vi "DIV_ACELTRS..vi"(5 "LIMITE MIN 2":dbl, 6 "LIMITE MAX 2":dbl, 7 "all rows":dbl[][](array[numeric])) -> (0 "concatenated string":string, 1 "ACELEROMETROS OK":bool)   [LabVIEW 2015]
panel:
  out "spreadsheet string":string
  out "Array 6":string[](array[string])
  out "transposed array":string[][](array[string])
  out "Array 5":string[](array[string])
  out "Array 4":string[][](array[string])
  out "Array 3":string[][](array[string])
  out "deleted portion 4":i32
  out "Array 2":string[][](array[string])
  out "Array":string[](array[string])
  out "deleted portion 3":i32
  out "Array 8":string[][](array[string])
  out "repet":i32
  out "FALLO ACELEROMETROS":string[][](array[string])
  out "BAJA SEÑAL 2":bool
  out "ACEL.SATURADO 2":bool
  out "deleted portion 2":i32
  out "deleted portion":i32
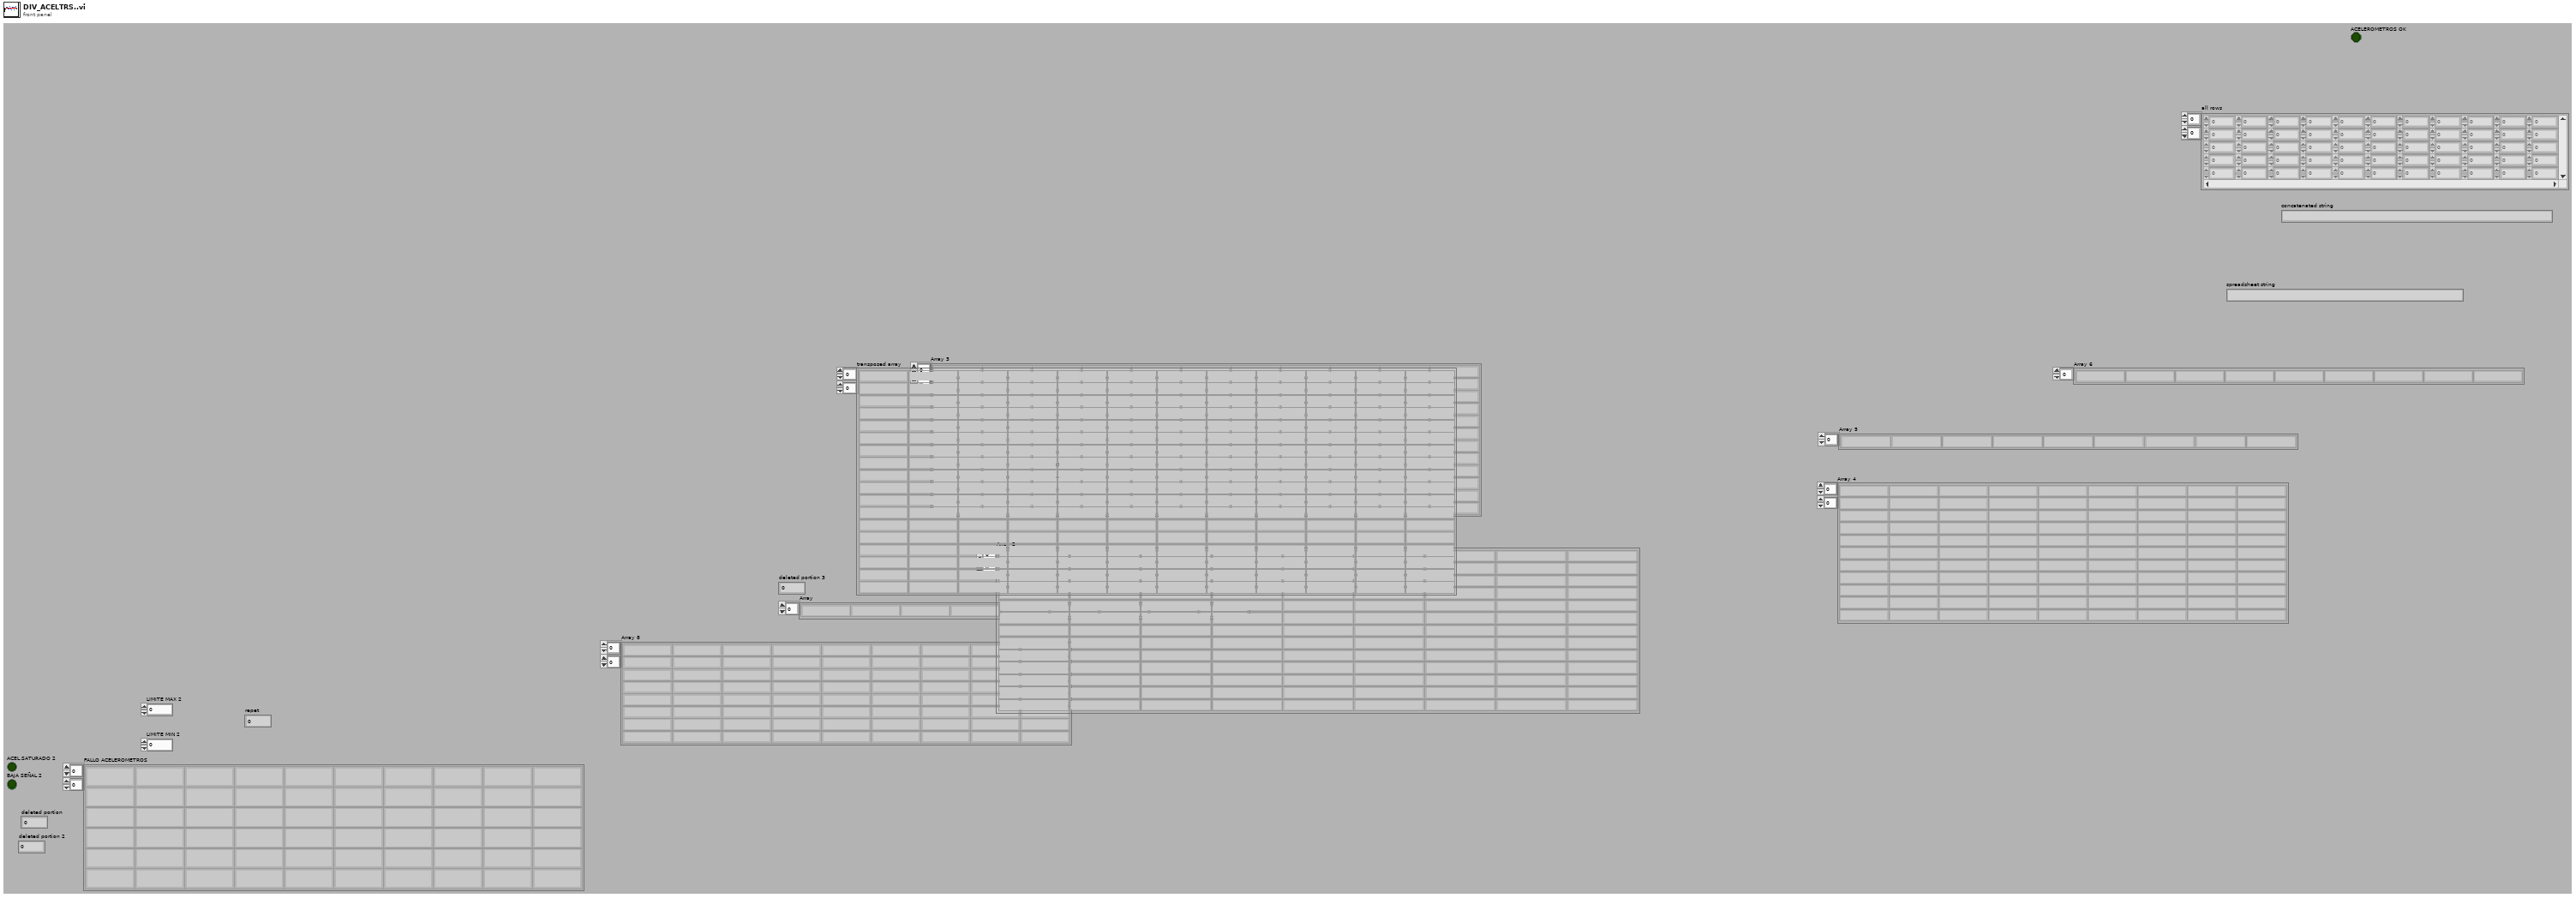
[diagram p1: front panel]
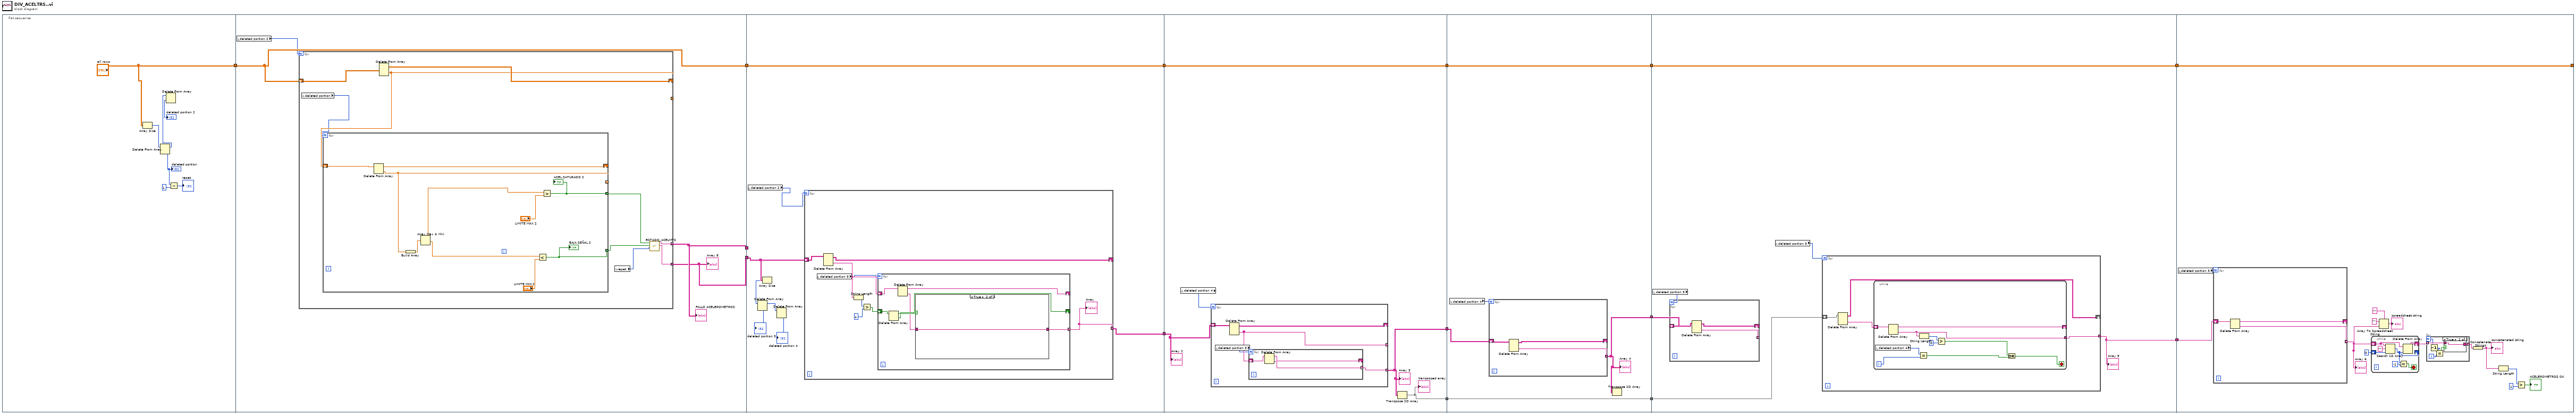
[diagram p0: block diagram]
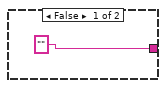
[diagram p2: hidden frame]
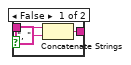
[diagram p3: hidden frame]
diagram:
  n1 = flat-sequence {
    tunnel: ["all rows"] -> w14
    tunnel: w14 -> [w25]
    tunnel: [w25] -> w13
    tunnel: [w23] -> w11
    tunnel: [w22] -> w10
    tunnel: w13 -> [w52]
    tunnel: [w52] -> w12
    tunnel: w11 -> [_]
    tunnel: w10 -> [w50]
    tunnel: [w47] -> w9
    tunnel: w12 -> [w74]
    tunnel: w9 -> [w73]
    tunnel: [w74] -> w8
    tunnel: [w71] -> w7
    tunnel: [w70] -> w3
    tunnel: w8 -> [w87]
    tunnel: w7 -> [w85]
    tunnel: [w87] -> w6
    tunnel: [w84] -> w5
    tunnel: [w83] -> w4
    tunnel: w3 -> [w83]
    tunnel: w6 -> [w96]
    tunnel: w5 -> [w94]
    tunnel: w4 -> [w92]
    tunnel: [w96] -> w2
    tunnel: [w91] -> w1
    tunnel: [w127] -> _
    tunnel: w2 -> [w127]
    tunnel: w1 -> [w125]
    frame #0 {
      n2 = Array Size(array="all rows") -> (size(s)=w21:i32[])
      n3 = Delete From Array(array=w21) -> (deleted portion=w18:i32, array with subset deleted=w19:i32[])  [unwired: 2 in]
      "deleted portion" <- w18
      n4 = Delete From Array(array=w19) -> (deleted portion=→"deleted portion 2":i32)  [unwired: 2 in, 1 out]
      n5 = Subtract(x=w18, y=1) -> (x-y=→"repet":i32)
    }
    frame #1 {
      n6 = local read "deleted portion 2"() -> (w24:i32)
      n7 = for {
        N: w24 -> [_]
        shift-right: [w33] -> _
        shift-left: w25 -> [w34]
        tunnel: [w32] -> _ mode=indexing
        tunnel: [w29] -> w23 mode=indexing
        tunnel: [w26] -> w22 mode=indexing
        n8 = local read "deleted portion"() -> (w28:i32)
        n9 = Delete From Array(array=w34) -> (deleted portion=w32:dbl[], array with subset deleted=w33:dbl[][])  [unwired: 3 in]
        n10 = for {
          N: w28 -> [_]
          shift-right: [w43] -> _
          shift-left: w32 -> [w44]
          tunnel: [w38] -> _ mode=indexing
          tunnel: [w36] -> w31 mode=indexing
          tunnel: [w35] -> w30 mode=indexing
          n11 = Delete From Array(array=w44) -> (deleted portion=w38:dbl, array with subset deleted=w43:dbl[])  [unwired: 2 in]
          n12 = Build Array(w38) -> (w37:dbl[])
          n13 = Array Max & Min(array=w37) -> (max value=w40:dbl, min value=w39:dbl)  [unwired: 2 out]
          n14 = Less?(x=w39, y="LIMITE MIN 2") -> (x < y?=w35:bool)
          "BAJA SEÑAL 2" <- w35
          n15 = Greater?(x=w40, y="LIMITE MAX 2") -> (0:w36:bool)
          "ACEL.SATURADO 2" <- w36
        }
        n16 = local read "repet"() -> (w27:i32)
        n17 = call "ESTADO_ACELMTS.vi"("Numeric"=w27, "Array 2"=w30, "Array"=w31) -> ("Array 8"=w26:string[], "Array 14"=w29:string[])  [unwired: 6 in]
      }
      "FALLO ACELEROMETROS" <- w23
      "Array 8" <- w22
    }
    frame #2 {
      n18 = local read "deleted portion 2"() -> (w51:i32)
      n19 = Array Size(array=w50) -> (size(s)=w49:i32[])
      n20 = Delete From Array(array=w49) -> (deleted portion=→"deleted portion 3":i32, array with subset deleted=w46:i32[])  [unwired: 2 in]
      n21 = Delete From Array(array=w46) -> (deleted portion=→"deleted portion 4":i32)  [unwired: 2 in, 1 out]
      n22 = for {
        N: w51 -> [_]
        shift-right: [w59] -> _
        shift-left: w50 -> [w60]
        tunnel: [w54] -> w47 mode=indexing
        n23 = local read "deleted portion 3"() -> (w53:i32)
        n24 = Delete From Array(array=w60) -> (deleted portion=w56:string[], array with subset deleted=w59:string[][])  [unwired: 3 in]
        n25 = String Length(string=w56) -> (length=w58:i32[])
        n26 = Greater?(x=w58, y=4) -> (0:w55:bool[])
        n27 = for {
          N: w53 -> [_]
          shift-right: [w64] -> _
          shift-left: w55 -> [w65]
          shift-right: [w66] -> _
          shift-left: w56 -> [w67]
          tunnel: [w61] -> w54 mode=indexing
          n28 = Delete From Array(array=w65) -> (deleted portion=w63:bool, array with subset deleted=w64:bool[])  [unwired: 2 in]
          n29 = Delete From Array(array=w67) -> (deleted portion=w62:string, array with subset deleted=w66:string[])  [unwired: 2 in]
          n30 = case shown="True" w63 {
            tunnel: w62 -> [_ w69]
            tunnel: ["" w69] -> w61
            frame False {
            }
            frame True {
            }
          }
        }
        "Array" <- w54
      }
    }
    frame #3 {
      n31 = local read "deleted portion 4"() -> (w72:i32)
      n32 = for {
        N: w72 -> [_]
        shift-right: [w78] -> _
        shift-left: w73 -> [w79]
        tunnel: [w77] -> _ mode=indexing
        tunnel: [w76] -> w71 mode=indexing
        n33 = local read "deleted portion 3"() -> (w75:i32)
        n34 = Delete From Array(array=w79) -> (deleted portion=w77:string[], array with subset deleted=w78:string[][])  [unwired: 3 in]
        n35 = for {
          N: w75 -> [_]
          shift-right: [w81] -> _
          shift-left: w77 -> [w82]
          tunnel: [w80] -> w76 mode=indexing
          n36 = Delete From Array(array=w82) -> (deleted portion=w80:string, array with subset deleted=w81:string[])  [unwired: 2 in]
        }
      }
      "Array 3" <- w71
      n37 = Transpose 2D Array(2D array=w71) -> (transposed array=w70:string[][])
      "transposed array" <- w70
      "Array 2" <- w73
    }
    frame #4 {
      n38 = local read "deleted portion 4"() -> (w86:i32)
      n39 = for {
        N: w86 -> [_]
        shift-right: [w89] -> _
        shift-left: w85 -> [w90]
        tunnel: [w88] -> w84 mode=indexing
        n40 = Delete From Array(array=w90) -> (deleted portion=w88:string[], array with subset deleted=w89:string[][])  [unwired: 3 in]
      }
      "Array 4" <- w84
      n41 = Transpose 2D Array(2D array=w84) -> ()  [unwired: 1 out]
    }
    frame #5 {
      n42 = local read "deleted portion 3"() -> (w93:i32)
      n43 = for {
        N: w93 -> [_]
        shift-right: [w98] -> _
        shift-left: w94 -> [w99]
        tunnel: [w97] -> _ mode=indexing
        n44 = Delete From Array(array=w99) -> (deleted portion=w97:string[], array with subset deleted=w98:string[][])  [unwired: 3 in]
      }
      n45 = local read "deleted portion 3"() -> (w95:i32)
      n46 = for {
        N: w95 -> [_]
        shift-right: [w102] -> _
        shift-left: w92 -> [w103]
        tunnel: [w100] -> w91 mode=indexing
        n47 = Delete From Array(array=w103) -> (deleted portion=w101:string[], array with subset deleted=w102:string[][])  [unwired: 3 in]
        n48 = while {
          shift-right: [w110] -> _
          shift-left: w101 -> [w111]
          tunnel: [w104] -> w100
          i -> [w112]
          stop <- w105 stop-if-true
          n49 = local read "deleted portion 4"() -> (w113:i32)
          n50 = Delete From Array(array=w111) -> (deleted portion=w104:string, array with subset deleted=w110:string[])  [unwired: 2 in]
          n51 = Equal?(x=w113, y=w112) -> (x = y?=w107:bool)
          n52 = String Length(string=w104) -> (length=w109:i32)
          n53 = Greater?(x=w109, y=0) -> (0:w106:bool)
          n54 = Or(x=w106, y=w107) -> (x .or. y?=w105:bool)
        }
      }
      "Array 5" <- w91
    }
    frame #6 {
      n55 = local read "deleted portion 3"() -> (w126:i32)
      n56 = for {
        N: w126 -> [_]
        shift-right: [w146] -> _
        shift-left: w125 -> [w147]
        tunnel: [w145] -> w120 mode=indexing
        n57 = Delete From Array(array=w147) -> (deleted portion=w145:string, array with subset deleted=w146:string[])  [unwired: 2 in]
      }
      "Array 6" <- w120
      n58 = while {
        shift-right: [w133] -> w119
        shift-left: w120 -> [w134]
        shift-right: [w129] -> _
        shift-left: 0 ("index of element") -> [w132]
        stop <- w128 stop-if-true
        n59 = Search 1D Array(1D array=w134, element="", start index (0)=w132) -> (index of element=w129:i32)
        n60 = Equal?(x=w129, y=-1) -> (x = y?=w128:bool)
        n61 = Delete From Array(array=w134, index=w129) -> (array with subset deleted=w133:string[])  [unwired: 1 in, 1 out]
      }
      n62 = Array To Spreadsheet String(delimiter (Tab)="", array=w120, 3:"" ("format string")) -> (spreadsheet string=→"spreadsheet string":string)
      n63 = for {
        N -> [w138]
        tunnel: w119 -> [w140] mode=indexing
        tunnel: [w139] -> w121 mode=indexing
        i -> [w136]
        n64 = Decrement(x=w138) -> (x-1=w137:i32)
        n65 = Equal?(x=w137, y=w136) -> (x = y?=w135:bool)
        n66 = case shown="True" w135 {
          tunnel: w140 -> [w143 w144]
          tunnel: [w141 w144] -> w139
          frame False {
            n67 = Concatenate Strings(w143, ", " ("string")) -> (w141:string)
          }
          frame True {
          }
        }
      }
      n68 = Concatenate Strings(w121) -> (w117:string)
      "concatenated string" <- w117
      n69 = String Length(string=w117) -> (length=w116:i32)
      n70 = Greater?(x=w116, y=1) -> (0:→"ACELEROMETROS OK":bool)
    }
  }
